vi "WaitEngine.vi"(3 "Wait Time (ms)":u32, 4 "Wait Command":T1=enum."Init") -> (1 "Elapsed?":bool)   [LabVIEW 2016]
uses:
  WaitVI/Wait Command.ctl
panel:
  out "elapsed time (ms)":i32
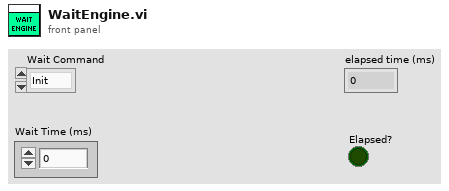
[diagram p1: front panel]
types:
  T1 = typedef "Wait Command.ctl" = enum16{"Running", "Init"}
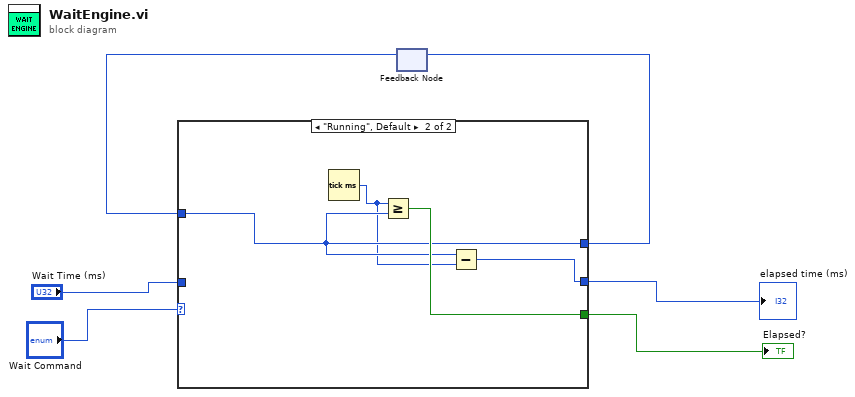
[diagram p0: block diagram]
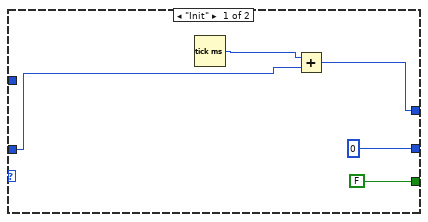
[diagram p2: hidden frame]
diagram:
  n1 = feedback #1() -> (w1:u32)  [unwired: 1 in]
  n2 = case shown="\"Running\", Default" "Wait Command" {
    tunnel: "Wait Time (ms)" -> [w7 _]
    tunnel: [FALSE w15] -> w5
    tunnel: [0 ("elapsed time (ms)") w12] -> w3
    tunnel: [w8 w14] -> w2
    tunnel: w1 -> [_ w14]
    frame "Init" {
      n3 = Tick Count (ms)() -> (millisecond timer value=w9:u32)
      n4 = Add(x=w9, y=w7) -> (x+y=w8:u32)
    }
    frame "Running", Default {
      n5 = Tick Count (ms)() -> (millisecond timer value=w13:u32)
      n6 = Greater Or Equal?(x=w13, y=w14) -> (x >= y?=w15:bool)
      n7 = Subtract(x=w14, y=w13) -> (x-y=w12:u32)
    }
  }
  "Elapsed?" <- w5
  "elapsed time (ms)" <- w3
  n8 = feedback-in #1(w2) -> ()
